vi "DMR_GetDevice.vi"(0 "search string IN":string="*", 1 "search mode IN":enum32{"by serial", "by family", "by product"}(ring), 2 "use device number as ID IN":bool, 3 "wildcard IN":string="*", 4 "device number IN":i32) -> (5 "device handle OUT":i32, 7 "error code OUT":i32)   [LabVIEW 2014]
doc: "Tries to locate a certain device in the system which matches the input criterias.\n\nThis function can be used to locate devices, which obey to criterias passed to the function.\n\nEXAMPLES:\n\nConsider three devices of sample device as installed in the current system. Their serial number may be 'SD00000001', 'SD00000002' and 'SD00000003', two devices are for grey video sources (product string 'SampleDevice-G), one for color source (product string 'SampleDevice-C').\n\nEach device has been assigned a unique ID, which is stored in the devices internal memory.\n\nSerial Product string device ID Family string\nSD00000001 SampleDevice-G 3 SampleDevice\nSD00000002 SampleDevice-C 66 SampleDevice\nSD00000003 SampleDevice-G 2 SampleDevice\n\nWhen now the serach mode is set to 'by serial', the search string input is set to 'SD0000*',\nthe device number stays 0 and the wildcard '*', this will find the first device whos serial number starts with 'SD0000' in the system( in this case device SD00000001 ).\n\nWhen instead of '0' '2' is passed as the device ID this will find the third device whos serial number starts with 'SD0000' in the system( in this case device SD00000003 ).\n\nIf now also the boolean input 'use device number as ID' is selected this will find the device whos serial number starts with 'SD0000' in the system which has a device ID of 2 stored in the device specifics internal memory( in this case again device SD00000003).\n\nSetting the search mode to 'by product' and the search string to 'SampleDevice-G' while setting the other inputs to their default values will find the first device whos product string is 'SampleDevice-G' in the system( in this case device SD00000001).\n\nBefore this VI can be used DMR_Init must have been called successfully.\n\nSee also:\nDMR_Init\n \nThe errorcode output will return 0 if successful or a negative error code otherwise. A list of valid error codes and their meaning can be found in the manual about this interface."
uses:
  mvDeviceManager.dll
panel:
  # "INPUT"
  # "OUTPUT"
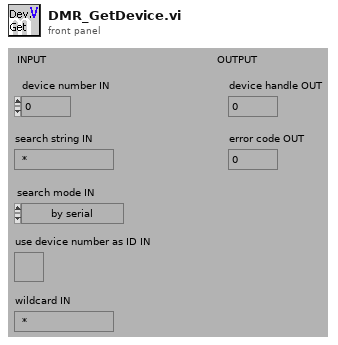
[diagram p1: front panel]
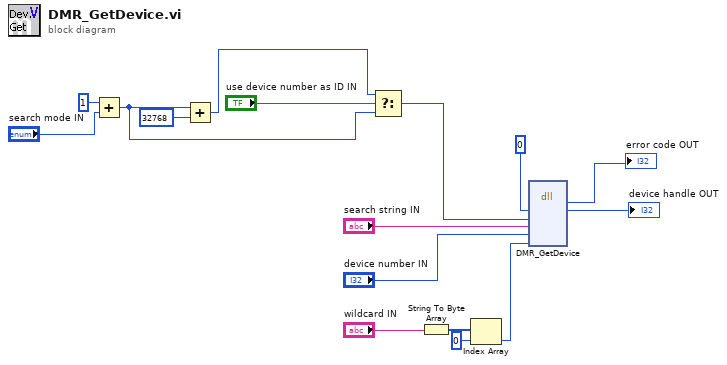
[diagram p0: block diagram]
diagram:
  n1 = Add(x=1, y="search mode IN") -> (x+y=w2:u32)
  n2 = Add(x=w2, y=u32 32768) -> (x+y=w1:u32)
  n3 = Select(t=w1, s="use device number as ID IN", f=w2) -> (s? t:f=w3:u32)
  n4 = String To Byte Array(string="wildcard IN") -> (unsigned byte array=w13:u8[])
  n5 = Index Array(array=w13, index=0 ("Index")) -> (element=w11:u8)
  n6 = dll-call lib="mvDeviceManager.dll" fn="DMR_GetDevice"("phDev"=0, "serarchMode"=w3, "serachString"="search string IN", "devNr"="device number IN", "wildcard"=w11) -> (→"error code OUT":i32, "phDev"=→"device handle OUT":i32)  [unwired: 7 in, 2 out]
